vi "Calculate Distance Point X to Y.vi"(1 "Y 2":dbl, 2 "X 2":dbl, 3 "Y 1":dbl, 4 "X 1":dbl) -> (0 "Distance":dbl)   [LabVIEW 2014, in "Position.lvclass"]
doc: "This VI calculates the distance from a point X to point Y on 2D XY plane."
uses:
  Position.lvclass
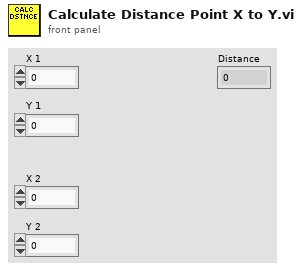
[diagram p1: front panel]
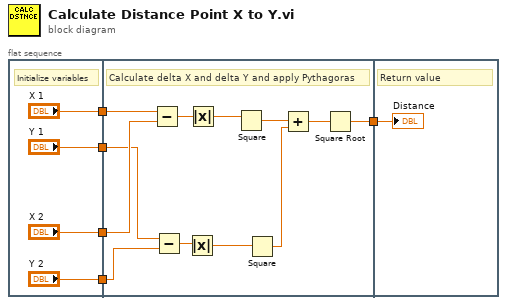
[diagram p0: block diagram]
diagram:
  n1 = flat-sequence {
    tunnel: ["X 1"] -> w5
    tunnel: ["Y 1"] -> w4
    tunnel: ["X 2"] -> w3
    tunnel: ["Y 2"] -> w2
    tunnel: w5 -> [w21]
    tunnel: w4 -> [w19]
    tunnel: w3 -> [w20]
    tunnel: w2 -> [w18]
    tunnel: [w14] -> w1
    tunnel: w1 -> [w22]
    frame #0 {
      # "Initialize variables"
    }
    frame #1 {
      # "Calculate delta X and delta Y and apply Pythagoras"
      n2 = Subtract(x=w21, y=w20) -> (x-y=w16:dbl)
      n3 = Subtract(x=w19, y=w18) -> (x-y=w17:dbl)
      n4 = Absolute Value(x=w17) -> (abs(x)=w12:dbl)
      n5 = Absolute Value(x=w16) -> (abs(x)=w13:dbl)
      n6 = Square(x=w13) -> (x^2=w11:dbl)
      n7 = Square(x=w12) -> (x^2=w10:dbl)
      n8 = Add(x=w11, y=w10) -> (x+y=w15:dbl)
      n9 = Square Root(x=w15) -> (sqrt(x)=w14:dbl)
    }
    frame #2 {
      # "Return value"
      "Distance" <- w22
    }
  }
